vi "Test Motors.vi"() -> ()   [LabVIEW 2013]
uses:
  <vilib>/robotics/Starter Kit/2.0/9632 Host Interface/NI_Robotics_Starter Kit Host_9632_2.0.lvclass
  <vilib>/robotics/Utilities/RPM to Radians per Second (Scalar).vi
  <vilib>/robotics/Utilities/Radians per Second to RPM (Scalar).vi
  <vilib>/robotics/Utilities/NI_Robotics Utilities.lvlib
  <vilib>/robotics/Starter Kit/Host Interface/NI_Robotics_Starter Kit Host.lvclass
panel:
  in  "数值":dbl
  in  "Left":dbl(slide) min=-100.0 max=100.0 step=4.0 scale=-70.0..70.0
  in  "Right":dbl(slide) min=-100.0 max=100.0 step=4.0 scale=-70.0..70.0
  out "Wheel Velocities (rpm)":cluster{"Left":dbl, dbl, "Right":dbl, dbl}(graph)
  in  "stop":bool
  # "Caution:  Moving the sliders will drive the robot.  Please ensure that it can safely move before continuing.\n\nTurn the MOTORS switch on, then move the sliders to control the forward wheel velocities in RPM."
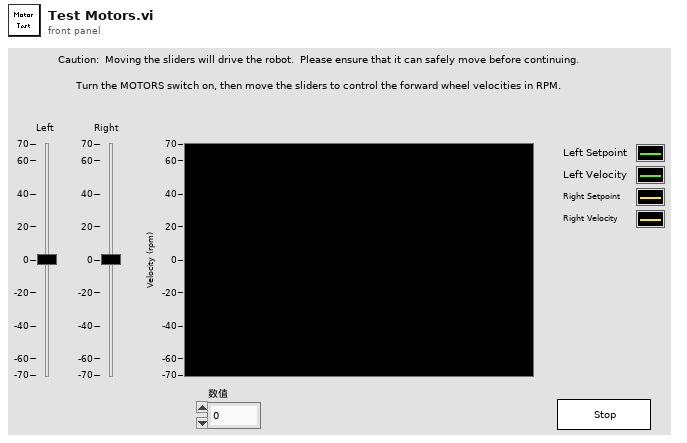
[diagram p1: front panel]
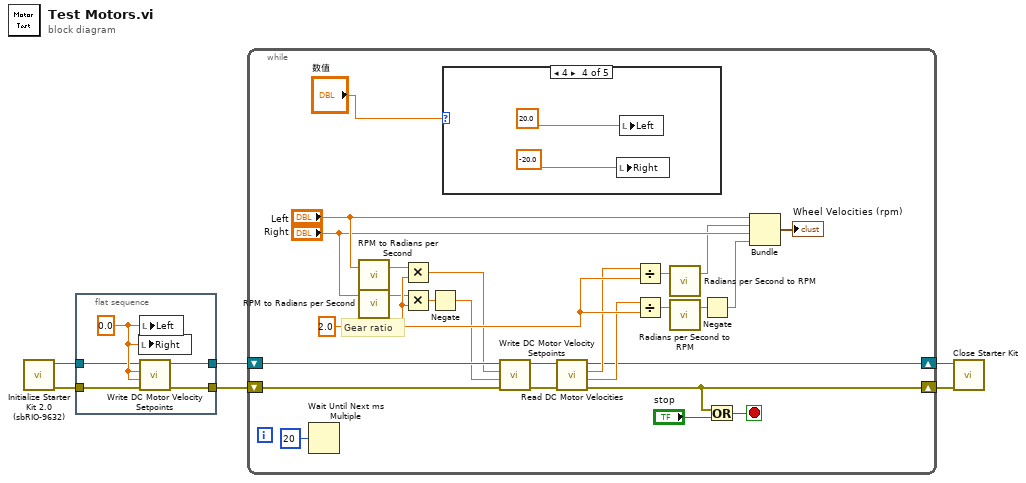
[diagram p0: block diagram]
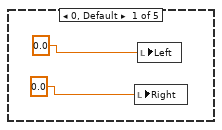
[diagram p2: hidden frame]
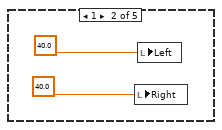
[diagram p3: hidden frame]
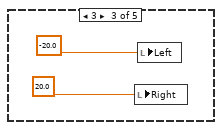
[diagram p4: hidden frame]
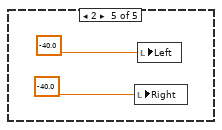
[diagram p5: hidden frame]
diagram:
  n1 = call <vilib>:"Initialize Starter Kit 2.0 (sbRIO-9632).vi"() -> ("error out"=w2:errorcluster, "FPGA starter kit host 2.0 out"=w1:refnum<class "NI_Robotics_Starter Kit Host_9632_2.0.lvclass">)  [unwired: 10 in]
  n2 = flat-sequence {
    tunnel: w1 -> [w10]
    tunnel: w2 -> [w7]
    tunnel: [w9] -> w6
    tunnel: [w8] -> w5
    frame #0 {
      w11 = 0.0 ("left ccw motor velocity (rad/s)")
      n3 = local write "Right"(w11) -> ()
      n4 = local write "Left"(w11) -> ()
      n5 = call <vilib>:"Write DC Motor Velocity Setpoints.vi"("error in (no error)"=w7, "right motor ccw velocity (rad/s)"=w11, "left motor ccw velocity (rad/s)"=w11, "starter kit host in"=w10) -> ("error out"=w8:errorcluster, "starter kit host out"=w9:refnum<class "NI_Robotics_Starter Kit Host_9632_2.0.lvclass">)  [unwired: 6 in]
    }
  }
  n6 = while {
    shift-right: [w13] -> w3
    shift-left: w5 -> [w19]
    shift-right: [w14] -> w4
    shift-left: w6 -> [w22]
    stop <- w37 stop-if-true
    w32 = 2.0 ("y")
    # "Gear ratio"
    n7 = Wait Until Next ms Multiple(millisecond multiple=u32 20) -> ()  [unwired: 1 out]
    n8 = call-poly <vilib>:"RPM to Radians per Second.vi"("rpm"="Left") -> ("radians per second"=w30:dbl)  [unwired: 2 in]
    n9 = call-poly <vilib>:"RPM to Radians per Second.vi"("rpm"="Right") -> ("radians per second"=w28:dbl)  [unwired: 2 in]
    n10 = Multiply(x=w30, y=w32) -> (x*y=w21:dbl)
    n11 = Multiply(x=w28, y=w32) -> (x*y=w34:dbl)
    n12 = Negate(x=w34) -> (-x=w20:dbl)
    n13 = case shown="4" "数值" {
      frame 0, Default {
        n14 = local write "Right"(0.0) -> ()
        n15 = local write "Left"(0.0) -> ()
      }
      frame 1 {
        n16 = local write "Right"(40.0) -> ()
        n17 = local write "Left"(40.0) -> ()
      }
      frame 3 {
        n18 = local write "Right"(20.0) -> ()
        n19 = local write "Left"(-20.0) -> ()
      }
      frame 4 {
        n20 = local write "Right"(-20.0) -> ()
        n21 = local write "Left"(20.0) -> ()
      }
      frame 2 {
        n22 = local write "Right"(-40.0) -> ()
        n23 = local write "Left"(-40.0) -> ()
      }
    }
    n24 = call <vilib>:"Write DC Motor Velocity Setpoints.vi"("error in (no error)"=w19, "right motor ccw velocity (rad/s)"=w20, "left motor ccw velocity (rad/s)"=w21, "starter kit host in"=w22) -> ("error out"=w15:errorcluster, "starter kit host out"=w16:refnum<class "NI_Robotics_Starter Kit Host_9632_2.0.lvclass">)  [unwired: 6 in]
    n25 = call <vilib>:"Read DC Motor Velocities.vi"("error in (no error)"=w15, "starter kit host in"=w16) -> ("error out"=w13:errorcluster, "right motor ccw velocity (rad/s)"=w17:dbl, "left motor ccw velocity (rad/s)"=w18:dbl, "starter kit host out"=w14:refnum<class "NI_Robotics_Starter Kit Host_9632_2.0.lvclass">)  [unwired: 6 in]
    n26 = Divide(x=w18, y=w32) -> (x/y=w27:dbl)
    n27 = Divide(x=w17, y=w32) -> (x/y=w26:dbl)
    n28 = call-poly <vilib>:"Radians per Second to RPM.vi"("radians per second"=w27) -> ("rpm"=w25:dbl)  [unwired: 2 in]
    n29 = call-poly <vilib>:"Radians per Second to RPM.vi"("radians per second"=w26) -> ("rpm"=w33:dbl)  [unwired: 2 in]
    n30 = Negate(x=w33) -> (-x=w24:dbl)
    n31 = Or(x=w13, y="stop") -> (x .or. y?=w37:bool)
    n32 = Bundle("Left"="Left", "rpm"=w25, "Right"="Right", w24) -> (→"Wheel Velocities (rpm)":cluster{"Left":dbl, "rpm":dbl, "Right":dbl, dbl})  [unwired: 1 in]
  }
  n33 = call-dynamic "Close Starter Kit.vi"("error in (no error)"=w3, "starter kit host in"=w4) -> ()  [unwired: 9 in, 1 out]
